vi "Set Echo Off.vi"() -> ()   [LabVIEW 2017]
panel:
  in  "VISA resource name":refnum<visa-resource-name>="COM1"
  out "VISA resource name out":refnum<visa-resource-name>
  out "error out":errorcluster
  in  "error in (no error)":errorcluster
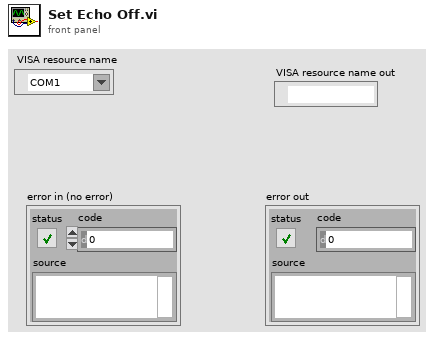
[diagram p1: front panel]
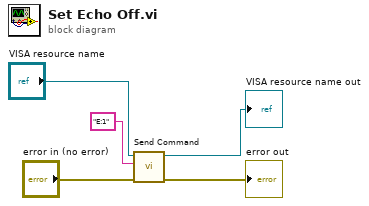
[diagram p0: block diagram]
diagram:
  n1 = call "Send Command.vi"("error in (no error)"="error in (no error)", "command"="E:1" ("query string"), "VISA resource name"="VISA resource name") -> ("error out"=→"error out":errorcluster, "VISA resource name out"=→"VISA resource name out":refnum<visa-resource-name>)  [unwired: 7 in]
